vi "Show Overview.vi"(11 "UI Data in":refnum<class "Settings UI.lvclass">) -> (3 "UI Data out":refnum<class "Settings UI.lvclass">)   [LabVIEW 2020, in "Output Sequencer.lvlib" / "Settings UI.lvclass"]
uses:
  Settings UI.lvclass
  Types/Tree Index Enum.ctl
  Settings UI.lvclass/Settings UI.ctl
  Globals/Global Tree Data.vi
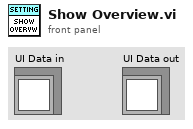
[diagram p1: front panel]
types:
  T1 = typedef "Output Sequencer.lvlib/Settings UI.lvclass/Tree Index Enum.ctl" = enum16{"General Settings", "Num Steps", "Num Analog", "Num Digital", "Show Confirmation", "Interp Priority", "Adv Timing", "Enable Conditions", "Seq Execution", "Reset Test Start", "Only When Test", "Delay After Test", "Start condition", "Re-triggering", "Stop condition", "Stop After Cycles", "Stop Values", "Default Values", "Default Analog", "Default Digital", "Steps", "Step #", "Description", "Precondition", "Duration", "Mode", "Delay Between Vals", "Analog Values", "Digital Values", "Postcondition", "On True", "On False"}
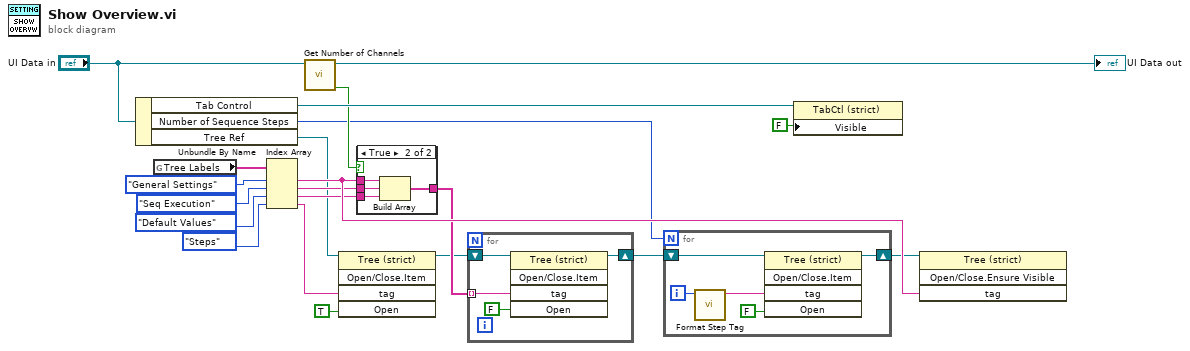
[diagram p0: block diagram]
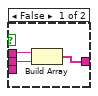
[diagram p2: hidden frame]
diagram:
  n1 = Unbundle By Name("UI Data in") -> ("Tab Control"=w17:refnum<vi>, "Number of Sequence Steps"=w2:i32, "Tree Ref"=w1:refnum<vi>)
  n2 = global read "Global Tree Data.vi" "Tree Labels"() -> (w7:string[])
  n3 = Index Array(array=w7, index #1=Tree_Index_Enum."General Settings" ("Tree Index Enum"), index #2=Tree_Index_Enum."Seq Execution" ("Tree Index Enum"), index #3=Tree_Index_Enum."Default Values" ("Tree Index Enum"), index #4=Tree_Index_Enum."Steps" ("Tree Index Enum")) -> (element #1=w19:string, element #2=w8:string, element #3=w9:string, element #4=w10:string)
  n4 = call "Get Number of Channels.vi"("UI Data In"="UI Data in") -> ("Channels Defined"=w11:bool, "UI Data out"=→"UI Data out":refnum<class "Settings UI.lvclass">)  [unwired: 7 in, 2 out]
  n5 = invoke on="Invoke Node" class="Tree (strict)" method="Open/Close.Item"(reference=w1, "tag"=w10, "Open"=TRUE ("Open?")) -> (reference out=w13:refnum<vi>)  [unwired: 2 in, 4 out]
  n6 = case shown="True" w11 {
    tunnel: w19 -> [w24 w28]
    tunnel: w9 -> [_ w26]
    tunnel: [w23 w27] -> w14
    tunnel: w8 -> [w22 w25]
    frame False {
      n7 = Build Array(w24, w22) -> (w23:string[])
    }
    frame True {
      n8 = Build Array(w28, w25, w26) -> (w27:string[])
    }
  }
  n9 = for {
    tunnel: w14 -> [w31] mode=indexing
    shift-right: [w29] -> w12
    shift-left: w13 -> [w30]
    n10 = invoke on="Invoke Node" class="Tree (strict)" method="Open/Close.Item"(reference=w30, "tag"=w31, "Open"=FALSE ("Open?")) -> (reference out=w29:refnum<vi>)  [unwired: 2 in, 4 out]
  }
  n11 = for {
    N: w2 -> [_]
    shift-right: [w35] -> w18
    shift-left: w12 -> [w36]
    i -> [w33]
    n12 = call "Format Step Tag.vi"("Step Number"=w33) -> ("Tag"=w34:string)  [unwired: 10 in]
    n13 = invoke on="Invoke Node" class="Tree (strict)" method="Open/Close.Item"(reference=w36, "tag"=w34, "Open"=FALSE ("Open?")) -> (reference out=w35:refnum<vi>)  [unwired: 2 in, 4 out]
  }
  n14 = property on="Property Node" class="TabCtl (strict)"(reference=w17, "Visible"=FALSE) -> ()  [unwired: 1 in, 2 out]
  n15 = invoke on="Invoke Node" class="Tree (strict)" method="Open/Close.Ensure Visible"(reference=w18, "tag"=w19) -> ()  [unwired: 2 in, 4 out]
